vi "Calib_Inst_ch_info.vi"(1 "Input string":string) -> (0 "instrument to calibrate":T1(array[cluster])=[{"high limit (10V)"=5.0, "low limit (-10V)"=3.0, "Ch No"=1, "Off ch no"=1}, {"high limit (10V)"=5.0, "low limit (-10V)"=3.0, "Ch No"=2, "Off ch no"=1}] {"Off ch no" min=0 max=1; "Ch No" min=0 max=7; "low limit (-10V)" min=-10 max=10 format="%.3f"; "high limit (10V)" min=-10 max=10 format="%.3f"})   [LabVIEW 2010]
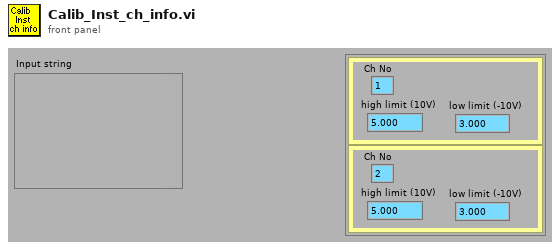
[diagram p1: front panel]
types:
  T1 = cluster{"high limit (10V)":sgl, "low limit (-10V)":sgl, "Ch No":i16, "Off ch no":i8}[]
  T2 = cluster{"high limit (10V)":sgl, "low limit (-10V)":sgl, "Ch No":i16, "Off ch no":i8}
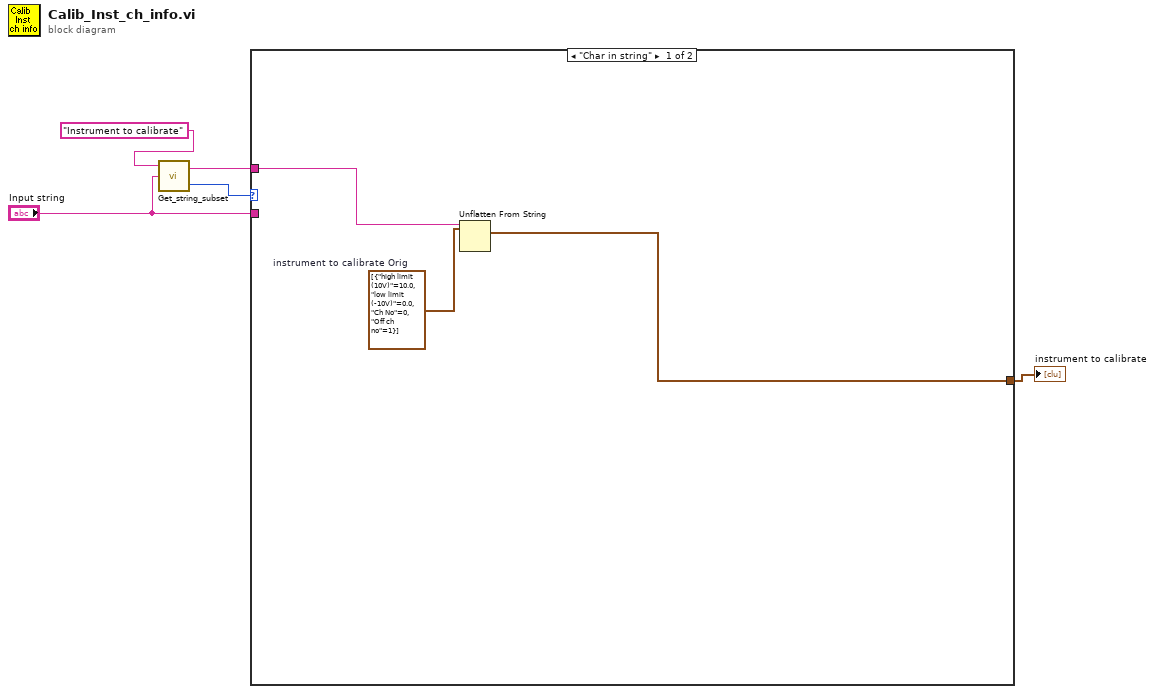
[diagram p0: block diagram]
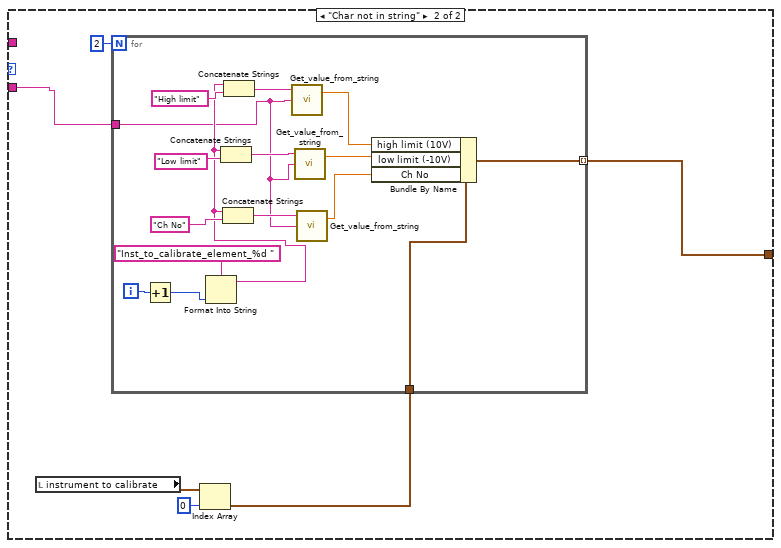
[diagram p2: hidden frame]
diagram:
  n1 = call "Get_string_subset.vi"("String to split"="Input string", "File Label"="Instrument to calibrate") -> ("Status"=w3:enum16{"Char in string", "Char not in string"}, "Output string"=w2:string)  [unwired: 2 in]
  n2 = case shown="\"Char in string\"" w3 {
    tunnel: "Input string" -> [_ w10]
    tunnel: w2 -> [w8 _]
    tunnel: [w7 w9] -> w1
    frame "Char in string" {
      w6 = T1 [{"high limit (10V)"=10.0, "low limit (-10V)"=0.0, "Ch No"=0, "Off ch no"=1}]  # instrument to calibrate Orig
      n3 = Unflatten From String(type=w6, binary string=w8) -> (value=w7:T1)  [unwired: 1 in, 4 out]
    }
    frame "Char not in string" {
      n4 = local read "instrument to calibrate"() -> (w13:T1)
      n5 = Index Array(array=w13, index=0) -> (element=w11:T2)
      n6 = for {
        N: 2 -> [_]
        tunnel: w11 -> [w23]
        tunnel: w10 -> [w19]
        tunnel: [w15] -> w9 mode=indexing
        i -> [w30]
        n7 = Increment(x=w30) -> (x+1=w26:i32)
        n8 = Format Into String(format string="Inst_to_calibrate_element_%d ", w26) -> (resulting string=w24:string)  [unwired: 2 in, 1 out]
        n9 = Concatenate Strings(w24, "Low limit") -> (w20:string)
        n10 = Concatenate Strings(w24, "Ch No") -> (w21:string)
        n11 = Concatenate Strings(w24, "High limit") -> (w22:string)
        n12 = call "Get_value_from_string.vi"("Input string"=w19, "Variable name"=w22) -> ("Value"=w18:dbl)  [unwired: 1 in, 1 out]
        n13 = call "Get_value_from_string.vi"("Input string"=w19, "Variable name"=w20) -> ("Value"=w17:dbl)  [unwired: 1 in, 1 out]
        n14 = call "Get_value_from_string.vi"("Input string"=w19, "Variable name"=w21) -> ("Value"=w16:dbl)  [unwired: 1 in, 1 out]
        n15 = Bundle By Name(cluster=w23, "high limit (10V)"=w18, "low limit (-10V)"=w17, "Ch No"=w16) -> (w15:T2)
      }
    }
  }
  "instrument to calibrate" <- w1
